vi "Concatenate_Length.vi"(0 "Eje X":i32, 5 "Eje Y":i32, 7 "Eje Z":i32, 11 "error in":errorcluster) -> (4 "EJE X":string, 6 "EJE Y":string, 8 "EJE Z":string, 15 "error out":errorcluster)   [LabVIEW 2021]
doc: "VI to concatenate a 0 when the lenght is less than 2"
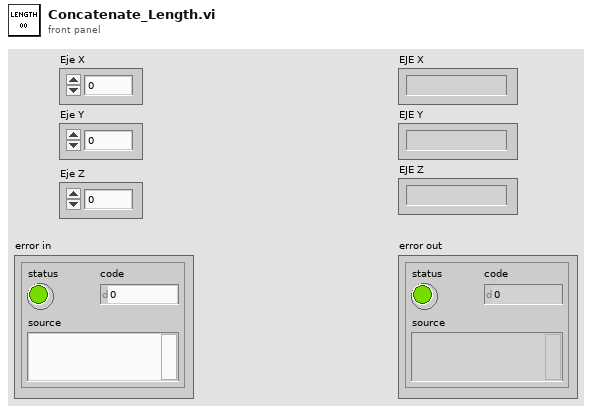
[diagram p1: front panel]
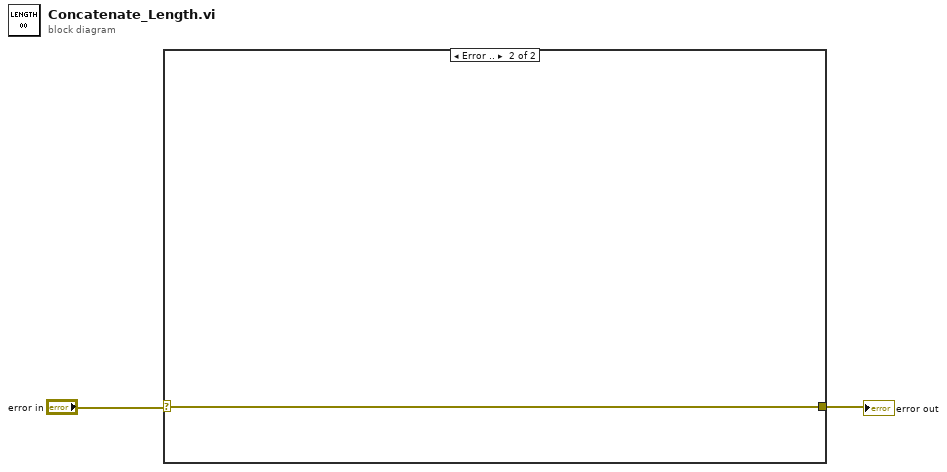
[diagram p0: block diagram]
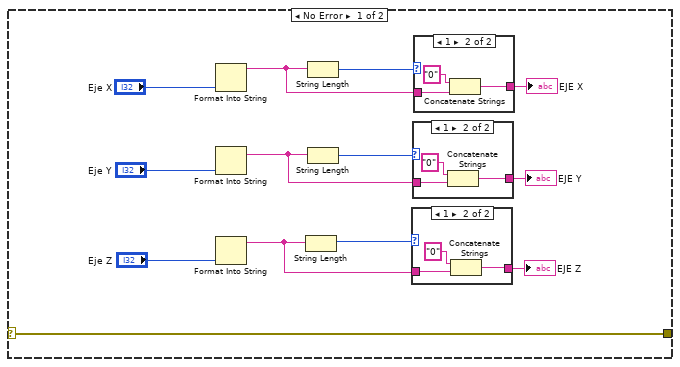
[diagram p2: hidden frame]
diagram:
  n1 = case shown="Error .." "error in" {
    selector: "error in" -> [w3 w28]
    tunnel: [w3 w28] -> w1
    frame No Error {
      n2 = Format Into String("Eje X") -> (resulting string=w9:string)  [unwired: 3 in, 1 out]
      n3 = Format Into String("Eje Y") -> (resulting string=w8:string)  [unwired: 3 in, 1 out]
      n4 = Format Into String("Eje Z") -> (resulting string=w7:string)  [unwired: 3 in, 1 out]
      n5 = String Length(string=w7) -> (length=w10:i32)
      n6 = String Length(string=w9) -> (length=w12:i32)
      n7 = String Length(string=w8) -> (length=w11:i32)
      n8 = case shown="1" w10 {
        tunnel: w7 -> [w16 w18]
        tunnel: [w16 w17] -> w4
        frame 2, Default {
        }
        frame 1 {
          n9 = Concatenate Strings("0" ("string"), w18) -> (w17:string)
        }
      }
      "EJE Z" <- w4
      n10 = case shown="1" w11 {
        tunnel: w8 -> [w20 w22]
        tunnel: [w20 w21] -> w5
        frame 2, Default {
        }
        frame 1 {
          n11 = Concatenate Strings("0" ("string"), w22) -> (w21:string)
        }
      }
      "EJE Y" <- w5
      n12 = case shown="1" w12 {
        tunnel: w9 -> [w24 w27]
        tunnel: [w24 w25] -> w6
        frame 2, Default {
        }
        frame 1 {
          n13 = Concatenate Strings("0" ("string"), w27) -> (w25:string)
        }
      }
      "EJE X" <- w6
    }
    frame Error {
    }
  }
  "error out" <- w1
